vi "Main_FPGA.vi"() -> ()   [LabVIEW 2017]
uses:
  <vilib>/eio/EIONode/EIONode.xnode
  <vilib>/rvi/eio/common/nirviEmuTemplateMethod_errors.vi
  <vilib>/rvi/DataTransferAndStorage/Container/XNode/niFpgaContainer.xnode
  <vilib>/rvi/interface/RandomDataEmulation/nirviRandomDataFpgaMultiElementTemplate.vi
  <vilib>/eio/EIOPropertyNode/EIOPropertyNode.xnode
  <vilib>/rvi/eio/common/nirviEmuTemplatePropertyGet_errors.vi
  <vilib>/rvi/eio/common/nirviEmuTemplatePropertyGet_noerrors.vi
  <vilib>/rvi/eio/common/nirviEmuTemplatePropertySet_errors.vi
  <vilib>/rvi/eio/common/nirviEmuTemplatePropertySet_noerrors.vi
  <vilib>/eio/EIOMethodNode/EIOMethodNode.xnode
  <vilib>/LabVIEW Targets/FPGA/cRIO/shared/nicrio_ModuleControls/nicrio_cRIO-9770_DataRatesRing.ctl
panel:
  out "Chassis Temperature":sgl
  in  "Tab Control":T1(tab)
  out "Data Over-Run 1":bool
  out "Error 1":errorcluster
  out "LO Frequency (Hz) 1":u32
  out "Downconverter Gain (dB) 1":fxp<+/-,15,8>
  out "PeakRFPower 1":fxp<+/-,12,8>
  in  "AcqSettings.Ch 1":T3={"Center Frequency (Hz)"=10000000, "Data Rate"=0, "Number of Samples"=1000, "Continuous"=FALSE, "Reference Level (dBm)"=0.0} {"Data Rate" items=["320.000 kS/s (NI 9770)", "256.000 kS/s (NI 9770)", "128.000 kS/s (NI 9770)", "64.000 kS/s (NI 9770)", "32.000 kS/s (NI 9770)", "16.000 kS/s (NI 9770)", "8.000 kS/s (NI 9770)", "4.000 kS/s (NI 9770)"]; "Center Frequency (Hz)" format="%.0p"}
  in  "Start 1":bool
  in  "Stop 1":bool
  in  "Start 2":bool
  in  "AcqSettings.Ch 2":T3={"Center Frequency (Hz)"=10000000, "Data Rate"=0, "Number of Samples"=1000, "Continuous"=FALSE, "Reference Level (dBm)"=0.0} {"Data Rate" items=["320.000 kS/s (NI 9770)", "256.000 kS/s (NI 9770)", "128.000 kS/s (NI 9770)", "64.000 kS/s (NI 9770)", "32.000 kS/s (NI 9770)", "16.000 kS/s (NI 9770)", "8.000 kS/s (NI 9770)", "4.000 kS/s (NI 9770)"]; "Center Frequency (Hz)" format="%.0p"}
  out "PeakRFPower 2":fxp<+/-,12,8>
  out "Data Over-Run 2":bool
  in  "Stop 2":bool
  out "Error 2":errorcluster
  out "LO Frequency (Hz) 2":u32
  out "Downconverter Gain (dB) 2":fxp<+/-,15,8>
  in  "Start 3":bool
  in  "AcqSettings.Ch 3":T3={"Center Frequency (Hz)"=10000000, "Data Rate"=0, "Number of Samples"=1000, "Continuous"=FALSE, "Reference Level (dBm)"=0.0} {"Data Rate" items=["320.000 kS/s (NI 9770)", "256.000 kS/s (NI 9770)", "128.000 kS/s (NI 9770)", "64.000 kS/s (NI 9770)", "32.000 kS/s (NI 9770)", "16.000 kS/s (NI 9770)", "8.000 kS/s (NI 9770)", "4.000 kS/s (NI 9770)"]; "Center Frequency (Hz)" format="%.0p"}
  out "PeakRFPower 3":fxp<+/-,12,8>
  out "Data Over-Run 3":bool
  in  "Stop 3":bool
  out "Error 3":errorcluster
  out "LO Frequency (Hz) 3":u32
  out "Downconverter Gain (dB) 3":fxp<+/-,15,8>
  in  "Start 4":bool
  in  "AcqSettings.Ch 4":T3={"Center Frequency (Hz)"=10000000, "Data Rate"=0, "Number of Samples"=1000, "Continuous"=FALSE, "Reference Level (dBm)"=0.0} {"Data Rate" items=["320.000 kS/s (NI 9770)", "256.000 kS/s (NI 9770)", "128.000 kS/s (NI 9770)", "64.000 kS/s (NI 9770)", "32.000 kS/s (NI 9770)", "16.000 kS/s (NI 9770)", "8.000 kS/s (NI 9770)", "4.000 kS/s (NI 9770)"]; "Center Frequency (Hz)" format="%.0p"}
  out "PeakRFPower 4":fxp<+/-,12,8>
  out "Data Over-Run 4":bool
  in  "Stop 4":bool
  out "Error 4":errorcluster
  out "LO Frequency (Hz) 4":u32
  out "Downconverter Gain (dB) 4":fxp<+/-,15,8>
  in  "Start 5":bool
  in  "AcqSettings.Ch 5":T3={"Center Frequency (Hz)"=10000000, "Data Rate"=0, "Number of Samples"=1000, "Continuous"=FALSE, "Reference Level (dBm)"=0.0} {"Data Rate" items=["320.000 kS/s (NI 9770)", "256.000 kS/s (NI 9770)", "128.000 kS/s (NI 9770)", "64.000 kS/s (NI 9770)", "32.000 kS/s (NI 9770)", "16.000 kS/s (NI 9770)", "8.000 kS/s (NI 9770)", "4.000 kS/s (NI 9770)"]; "Center Frequency (Hz)" format="%.0p"}
  out "PeakRFPower 5":fxp<+/-,12,8>
  out "Data Over-Run 5":bool
  in  "Stop 5":bool
  out "Error 5":errorcluster
  out "LO Frequency (Hz) 5":u32
  out "Downconverter Gain (dB) 5":fxp<+/-,15,8>
  in  "Start 6":bool
  in  "AcqSettings.Ch 6":T3={"Center Frequency (Hz)"=10000000, "Data Rate"=0, "Number of Samples"=1000, "Continuous"=FALSE, "Reference Level (dBm)"=0.0} {"Data Rate" items=["320.000 kS/s (NI 9770)", "256.000 kS/s (NI 9770)", "128.000 kS/s (NI 9770)", "64.000 kS/s (NI 9770)", "32.000 kS/s (NI 9770)", "16.000 kS/s (NI 9770)", "8.000 kS/s (NI 9770)", "4.000 kS/s (NI 9770)"]; "Center Frequency (Hz)" format="%.0p"}
  out "PeakRFPower 6":fxp<+/-,12,8>
  out "Data Over-Run 6":bool
  in  "Stop 6":bool
  out "Error 6":errorcluster
  out "LO Frequency (Hz) 6":u32
  out "Downconverter Gain (dB) 6":fxp<+/-,15,8>
  in  "Start 7":bool
  in  "AcqSettings.Ch 7":T3={"Center Frequency (Hz)"=10000000, "Data Rate"=0, "Number of Samples"=1000, "Continuous"=FALSE, "Reference Level (dBm)"=0.0} {"Data Rate" items=["320.000 kS/s (NI 9770)", "256.000 kS/s (NI 9770)", "128.000 kS/s (NI 9770)", "64.000 kS/s (NI 9770)", "32.000 kS/s (NI 9770)", "16.000 kS/s (NI 9770)", "8.000 kS/s (NI 9770)", "4.000 kS/s (NI 9770)"]; "Center Frequency (Hz)" format="%.0p"}
  out "PeakRFPower 7":fxp<+/-,12,8>
  out "Data Over-Run 7":bool
  in  "Stop 7":bool
  out "Error 7":errorcluster
  out "LO Frequency (Hz) 7":u32
  out "Downconverter Gain (dB) 7":fxp<+/-,15,8>
  in  "Start 8":bool
  in  "AcqSettings.Ch 8":T3={"Center Frequency (Hz)"=10000000, "Data Rate"=0, "Number of Samples"=1000, "Continuous"=FALSE, "Reference Level (dBm)"=0.0} {"Data Rate" items=["320.000 kS/s (NI 9770)", "256.000 kS/s (NI 9770)", "128.000 kS/s (NI 9770)", "64.000 kS/s (NI 9770)", "32.000 kS/s (NI 9770)", "16.000 kS/s (NI 9770)", "8.000 kS/s (NI 9770)", "4.000 kS/s (NI 9770)"]; "Center Frequency (Hz)" format="%.0p"}
  out "PeakRFPower 8":fxp<+/-,12,8>
  out "Data Over-Run 8":bool
  in  "Stop 8":bool
  out "Error 8":errorcluster
  out "LO Frequency (Hz) 8":u32
  out "Downconverter Gain (dB) 8":fxp<+/-,15,8>
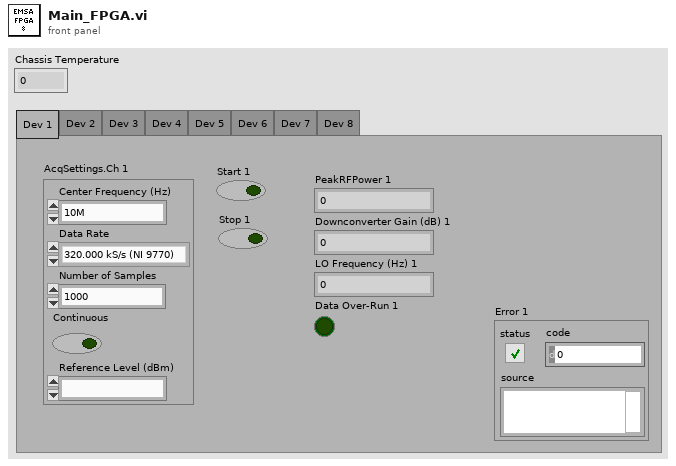
[diagram p1: front panel]
types:
  T1 = enum32{"Dev 1", "Dev 2", "Dev 3", "Dev 4", "Dev 5", "Dev 6", "Dev 7", "Dev 8"}
  T2 = typedef "nicrio_cRIO-9770_DataRatesRing.ctl" = u8
  T3 = cluster{"Center Frequency (Hz)":u32, "Data Rate":T2, "Number of Samples":i32, "Continuous":bool, "Reference Level (dBm)":fxp<+/-,14,7>}
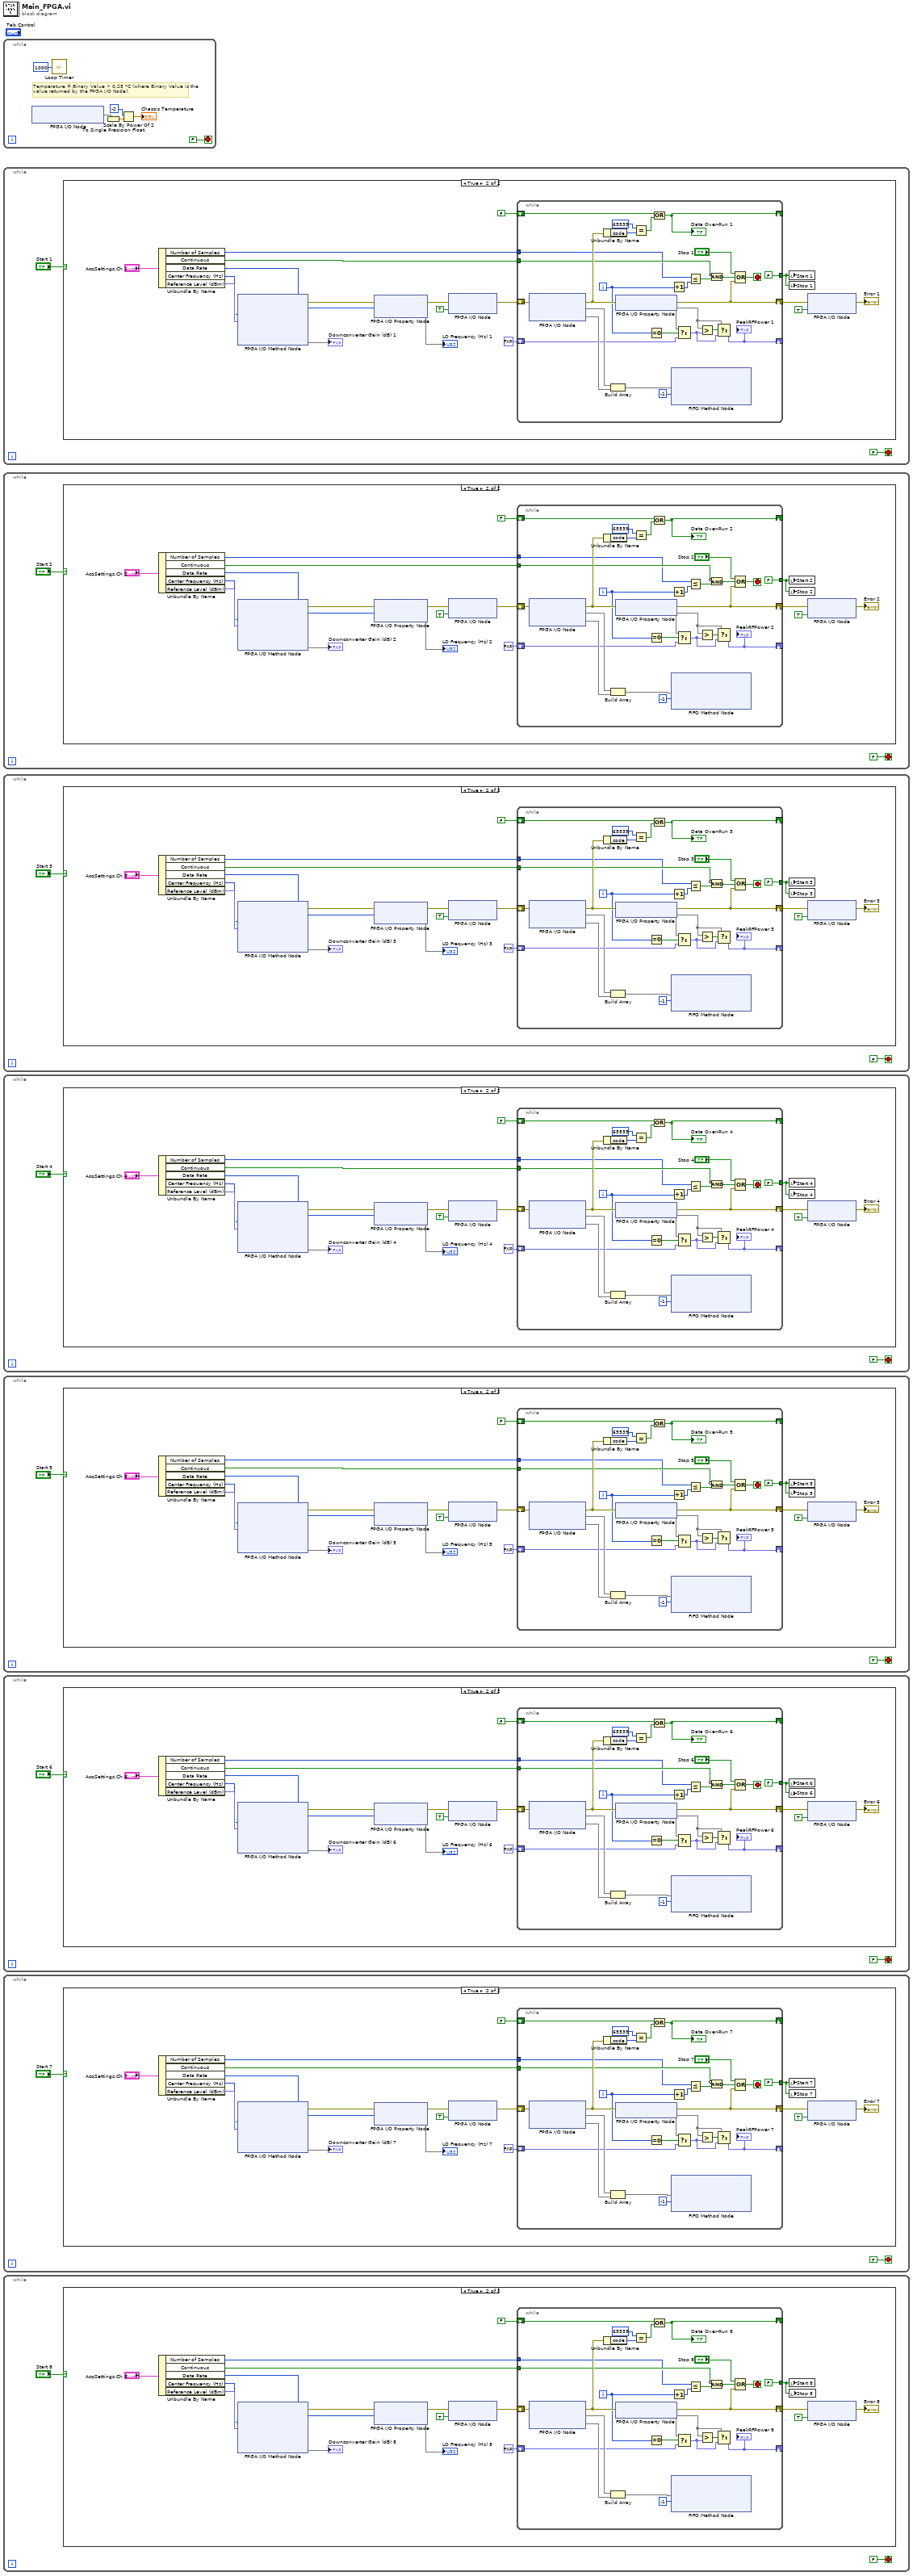
[diagram p0: block diagram]
diagram:
  n1 = while {
    stop <- FALSE stop-if-true
    # "Temperature = Binary Value × 0.25 °C (where Binary Value is the value returned by the FPGA I/O Node)."
    n2 = xnode "FPGA I/O Node"() -> ("Chassis Temperature"=w4)  [unwired: 1 in, 1 out]
    n3 = call "Loop Timer"("Count(mSec)"=u32 1000) -> ()  [unwired: 1 out]
    n4 = To Single Precision Float(number=w4) -> (single precision float=w6:sgl)
    n5 = Scale By Power Of 2(n=i16 -2, x=w6) -> (x*2^n=→"Chassis Temperature":sgl)
  }
  n6 = while {
    stop <- FALSE stop-if-true
    n7 = case shown="True" "Start 1" {
      frame False {
      }
      frame True {
        n8 = Unbundle By Name("AcqSettings.Ch 1") -> ("Number of Samples"=w10:i32, "Continuous"=w14:bool, "Data Rate"=w13:T2, "Center Frequency (Hz)"=w15:u32, "Reference Level (dBm)"=w16:fxp<+/-,14,7>)
        n9 = xnode "FPGA I/O Method Node"("Center Frequency"=w15, "Reference Level"=w16) -> ("error out"=w20:errorcluster, "Downconverter Gain"=→"Downconverter Gain (dB) 1")  [unwired: 4 in, 1 out]
        n10 = xnode "FPGA I/O Property Node"("error in"=w20, "Data Rate"=w13) -> ("error out"=w22:errorcluster, "LO Frequency"=→"LO Frequency (Hz) 1")  [unwired: 1 in, 1 out]
        n11 = xnode "FPGA I/O Node"("error in"=w22, "Mod1/Start"=TRUE ("start")) -> ("error out"=w21:errorcluster)  [unwired: 1 in, 1 out]
        n12 = while {
          shift-right: [w45] -> w25
          shift-left: w21 -> [w53]
          tunnel: [FALSE] -> w9
          shift-right: [w38] -> _
          shift-left: FALSE ("stop") -> [w40]
          shift-right: [w36] -> _
          shift-left: fxp<+/-,12,8> 0.0 ("Peak RF In Power") -> [w29]
          tunnel: w14 -> [w33]
          tunnel: w10 -> [w27]
          i -> [w31]
          stop <- w46 stop-if-true
          n13 = xnode "FPGA I/O Node"("error in"=w53) -> ("error out"=w43:errorcluster, "Mod1/RF In/I"=w52, "Mod1/RF In/Q"=w51)  [unwired: 2 in, 2 out]
          n14 = Unbundle By Name(w43) -> ("code"=w42:i32)
          n15 = Build Array(w52, w51) -> (w50:void[])
          n16 = xnode "FPGA I/O Property Node"("error in"=w43) -> ("error out"=w45:errorcluster, "Peak RF In Power"=w30)  [unwired: 1 in, 1 out]
          n17 = Equal?(x=65539, y=w42) -> (x = y?=w39:bool)
          n18 = Equal To 0?(x=w31) -> (x = 0?=w32:bool)
          n19 = Compound Arithmetic op=OR(w40, w39) -> (w38:bool)
          "Data Over-Run 1" <- w38
          n20 = xnode ("FIFO Method Node")("Element"=w50, "Timeout"=-1) -> ()  [unwired: 1 in, 2 out]
          n21 = Increment(x=w31) -> (x+1=w48:i32)
          n22 = Select(t=w30, s=w32, f=w29) -> (s? t:f=w28:fxp<+/-,12,8>)
          n23 = Less Or Equal?(x=w27, y=w48) -> (x <= y?=w35:bool)
          n24 = Greater?(x=w30, y=w28) -> (0:w37:bool)
          n25 = Compound Arithmetic op=AND(invert w33, w35) -> (w34:bool)
          n26 = Select(t=w30, s=w37, f=w28) -> (s? t:f=w36:fxp<+/-,12,8>)
          "PeakRFPower 1" <- w36
          n27 = Compound Arithmetic op=OR("Stop 1", w34, w45) -> (w46:bool)
        }
        n28 = local write "Start 1"(w9) -> ()
        n29 = local write "Stop 1"(w9) -> ()
        n30 = xnode "FPGA I/O Node"("error in"=w25, "Mod1/Stop"=TRUE ("stop")) -> ("error out"=→"Error 1":errorcluster)  [unwired: 1 in, 1 out]
      }
    }
  }
  n31 = while {
    stop <- FALSE stop-if-true
    n32 = case shown="True" "Start 2" {
      frame False {
      }
      frame True {
        n33 = Unbundle By Name("AcqSettings.Ch 2") -> ("Number of Samples"=w57:i32, "Continuous"=w61:bool, "Data Rate"=w60:T2, "Center Frequency (Hz)"=w62:u32, "Reference Level (dBm)"=w63:fxp<+/-,14,7>)
        n34 = xnode "FPGA I/O Method Node"("Center Frequency"=w62, "Reference Level"=w63) -> ("error out"=w67:errorcluster, "Downconverter Gain"=→"Downconverter Gain (dB) 2")  [unwired: 4 in, 1 out]
        n35 = xnode "FPGA I/O Property Node"("error in"=w67, "Data Rate"=w60) -> ("error out"=w69:errorcluster, "LO Frequency"=→"LO Frequency (Hz) 2")  [unwired: 1 in, 1 out]
        n36 = xnode "FPGA I/O Node"("error in"=w69, "Mod2/Start"=TRUE ("start")) -> ("error out"=w68:errorcluster)  [unwired: 1 in, 1 out]
        n37 = while {
          shift-right: [w92] -> w72
          shift-left: w68 -> [w100]
          tunnel: [FALSE] -> w56
          shift-right: [w85] -> _
          shift-left: FALSE ("stop") -> [w87]
          shift-right: [w83] -> _
          shift-left: fxp<+/-,12,8> 0.0 ("Peak RF In Power") -> [w76]
          tunnel: w61 -> [w80]
          tunnel: w57 -> [w74]
          i -> [w78]
          stop <- w93 stop-if-true
          n38 = xnode "FPGA I/O Node"("error in"=w100) -> ("error out"=w90:errorcluster, "Mod2/RF In/I"=w99, "Mod2/RF In/Q"=w98)  [unwired: 2 in, 2 out]
          n39 = Unbundle By Name(w90) -> ("code"=w89:i32)
          n40 = Build Array(w99, w98) -> (w97:void[])
          n41 = xnode "FPGA I/O Property Node"("error in"=w90) -> ("error out"=w92:errorcluster, "Peak RF In Power"=w77)  [unwired: 1 in, 1 out]
          n42 = Equal?(x=65539, y=w89) -> (x = y?=w86:bool)
          n43 = Equal To 0?(x=w78) -> (x = 0?=w79:bool)
          n44 = Compound Arithmetic op=OR(w87, w86) -> (w85:bool)
          "Data Over-Run 2" <- w85
          n45 = xnode ("FIFO Method Node")("Element"=w97, "Timeout"=-1) -> ()  [unwired: 1 in, 2 out]
          n46 = Increment(x=w78) -> (x+1=w95:i32)
          n47 = Select(t=w77, s=w79, f=w76) -> (s? t:f=w75:fxp<+/-,12,8>)
          n48 = Less Or Equal?(x=w74, y=w95) -> (x <= y?=w82:bool)
          n49 = Greater?(x=w77, y=w75) -> (0:w84:bool)
          n50 = Compound Arithmetic op=AND(invert w80, w82) -> (w81:bool)
          n51 = Select(t=w77, s=w84, f=w75) -> (s? t:f=w83:fxp<+/-,12,8>)
          "PeakRFPower 2" <- w83
          n52 = Compound Arithmetic op=OR("Stop 2", w81, w92) -> (w93:bool)
        }
        n53 = local write "Start 2"(w56) -> ()
        n54 = local write "Stop 2"(w56) -> ()
        n55 = xnode "FPGA I/O Node"("error in"=w72, "Mod2/Stop"=TRUE ("stop")) -> ("error out"=→"Error 2":errorcluster)  [unwired: 1 in, 1 out]
      }
    }
  }
  n56 = while {
    stop <- FALSE stop-if-true
    n57 = case shown="True" "Start 3" {
      frame False {
      }
      frame True {
        n58 = Unbundle By Name("AcqSettings.Ch 3") -> ("Number of Samples"=w104:i32, "Continuous"=w108:bool, "Data Rate"=w107:T2, "Center Frequency (Hz)"=w109:u32, "Reference Level (dBm)"=w110:fxp<+/-,14,7>)
        n59 = xnode "FPGA I/O Method Node"("Center Frequency"=w109, "Reference Level"=w110) -> ("error out"=w114:errorcluster, "Downconverter Gain"=→"Downconverter Gain (dB) 3")  [unwired: 4 in, 1 out]
        n60 = xnode "FPGA I/O Property Node"("error in"=w114, "Data Rate"=w107) -> ("error out"=w116:errorcluster, "LO Frequency"=→"LO Frequency (Hz) 3")  [unwired: 1 in, 1 out]
        n61 = xnode "FPGA I/O Node"("error in"=w116, "Mod3/Start"=TRUE ("start")) -> ("error out"=w115:errorcluster)  [unwired: 1 in, 1 out]
        n62 = while {
          shift-right: [w139] -> w119
          shift-left: w115 -> [w147]
          tunnel: [FALSE] -> w103
          shift-right: [w132] -> _
          shift-left: FALSE ("stop") -> [w134]
          shift-right: [w130] -> _
          shift-left: fxp<+/-,12,8> 0.0 ("Peak RF In Power") -> [w123]
          tunnel: w108 -> [w127]
          tunnel: w104 -> [w121]
          i -> [w125]
          stop <- w140 stop-if-true
          n63 = xnode "FPGA I/O Node"("error in"=w147) -> ("error out"=w137:errorcluster, "Mod3/RF In/I"=w146, "Mod3/RF In/Q"=w145)  [unwired: 2 in, 2 out]
          n64 = Unbundle By Name(w137) -> ("code"=w136:i32)
          n65 = Build Array(w146, w145) -> (w144:void[])
          n66 = xnode "FPGA I/O Property Node"("error in"=w137) -> ("error out"=w139:errorcluster, "Peak RF In Power"=w124)  [unwired: 1 in, 1 out]
          n67 = Equal?(x=65539, y=w136) -> (x = y?=w133:bool)
          n68 = Equal To 0?(x=w125) -> (x = 0?=w126:bool)
          n69 = Compound Arithmetic op=OR(w134, w133) -> (w132:bool)
          "Data Over-Run 3" <- w132
          n70 = xnode ("FIFO Method Node")("Element"=w144, "Timeout"=-1) -> ()  [unwired: 1 in, 2 out]
          n71 = Increment(x=w125) -> (x+1=w142:i32)
          n72 = Select(t=w124, s=w126, f=w123) -> (s? t:f=w122:fxp<+/-,12,8>)
          n73 = Less Or Equal?(x=w121, y=w142) -> (x <= y?=w129:bool)
          n74 = Greater?(x=w124, y=w122) -> (0:w131:bool)
          n75 = Compound Arithmetic op=AND(invert w127, w129) -> (w128:bool)
          n76 = Select(t=w124, s=w131, f=w122) -> (s? t:f=w130:fxp<+/-,12,8>)
          "PeakRFPower 3" <- w130
          n77 = Compound Arithmetic op=OR("Stop 3", w128, w139) -> (w140:bool)
        }
        n78 = local write "Start 3"(w103) -> ()
        n79 = local write "Stop 3"(w103) -> ()
        n80 = xnode "FPGA I/O Node"("error in"=w119, "Mod3/Stop"=TRUE ("stop")) -> ("error out"=→"Error 3":errorcluster)  [unwired: 1 in, 1 out]
      }
    }
  }
  n81 = while {
    stop <- FALSE stop-if-true
    n82 = case shown="True" "Start 4" {
      frame False {
      }
      frame True {
        n83 = Unbundle By Name("AcqSettings.Ch 4") -> ("Number of Samples"=w151:i32, "Continuous"=w155:bool, "Data Rate"=w154:T2, "Center Frequency (Hz)"=w156:u32, "Reference Level (dBm)"=w157:fxp<+/-,14,7>)
        n84 = xnode "FPGA I/O Method Node"("Center Frequency"=w156, "Reference Level"=w157) -> ("error out"=w161:errorcluster, "Downconverter Gain"=→"Downconverter Gain (dB) 4")  [unwired: 4 in, 1 out]
        n85 = xnode "FPGA I/O Property Node"("error in"=w161, "Data Rate"=w154) -> ("error out"=w163:errorcluster, "LO Frequency"=→"LO Frequency (Hz) 4")  [unwired: 1 in, 1 out]
        n86 = xnode "FPGA I/O Node"("error in"=w163, "Mod4/Start"=TRUE ("start")) -> ("error out"=w162:errorcluster)  [unwired: 1 in, 1 out]
        n87 = while {
          shift-right: [w186] -> w166
          shift-left: w162 -> [w194]
          tunnel: [FALSE] -> w150
          shift-right: [w179] -> _
          shift-left: FALSE ("stop") -> [w181]
          shift-right: [w177] -> _
          shift-left: fxp<+/-,12,8> 0.0 ("Peak RF In Power") -> [w170]
          tunnel: w155 -> [w174]
          tunnel: w151 -> [w168]
          i -> [w172]
          stop <- w187 stop-if-true
          n88 = xnode "FPGA I/O Node"("error in"=w194) -> ("error out"=w184:errorcluster, "Mod4/RF In/I"=w193, "Mod4/RF In/Q"=w192)  [unwired: 2 in, 2 out]
          n89 = Unbundle By Name(w184) -> ("code"=w183:i32)
          n90 = Build Array(w193, w192) -> (w191:void[])
          n91 = xnode "FPGA I/O Property Node"("error in"=w184) -> ("error out"=w186:errorcluster, "Peak RF In Power"=w171)  [unwired: 1 in, 1 out]
          n92 = Equal?(x=65539, y=w183) -> (x = y?=w180:bool)
          n93 = Equal To 0?(x=w172) -> (x = 0?=w173:bool)
          n94 = Compound Arithmetic op=OR(w181, w180) -> (w179:bool)
          "Data Over-Run 4" <- w179
          n95 = xnode ("FIFO Method Node")("Element"=w191, "Timeout"=-1) -> ()  [unwired: 1 in, 2 out]
          n96 = Increment(x=w172) -> (x+1=w189:i32)
          n97 = Select(t=w171, s=w173, f=w170) -> (s? t:f=w169:fxp<+/-,12,8>)
          n98 = Less Or Equal?(x=w168, y=w189) -> (x <= y?=w176:bool)
          n99 = Greater?(x=w171, y=w169) -> (0:w178:bool)
          n100 = Compound Arithmetic op=AND(invert w174, w176) -> (w175:bool)
          n101 = Select(t=w171, s=w178, f=w169) -> (s? t:f=w177:fxp<+/-,12,8>)
          "PeakRFPower 4" <- w177
          n102 = Compound Arithmetic op=OR("Stop 4", w175, w186) -> (w187:bool)
        }
        n103 = local write "Start 4"(w150) -> ()
        n104 = local write "Stop 4"(w150) -> ()
        n105 = xnode "FPGA I/O Node"("error in"=w166, "Mod4/Stop"=TRUE ("stop")) -> ("error out"=→"Error 4":errorcluster)  [unwired: 1 in, 1 out]
      }
    }
  }
  n106 = while {
    stop <- FALSE stop-if-true
    n107 = case shown="True" "Start 5" {
      frame False {
      }
      frame True {
        n108 = Unbundle By Name("AcqSettings.Ch 5") -> ("Number of Samples"=w198:i32, "Continuous"=w202:bool, "Data Rate"=w201:T2, "Center Frequency (Hz)"=w203:u32, "Reference Level (dBm)"=w204:fxp<+/-,14,7>)
        n109 = xnode "FPGA I/O Method Node"("Center Frequency"=w203, "Reference Level"=w204) -> ("error out"=w208:errorcluster, "Downconverter Gain"=→"Downconverter Gain (dB) 5")  [unwired: 4 in, 1 out]
        n110 = xnode "FPGA I/O Property Node"("error in"=w208, "Data Rate"=w201) -> ("error out"=w210:errorcluster, "LO Frequency"=→"LO Frequency (Hz) 5")  [unwired: 1 in, 1 out]
        n111 = xnode "FPGA I/O Node"("error in"=w210, "Mod5/Start"=TRUE ("start")) -> ("error out"=w209:errorcluster)  [unwired: 1 in, 1 out]
        n112 = while {
          shift-right: [w233] -> w213
          shift-left: w209 -> [w241]
          tunnel: [FALSE] -> w197
          shift-right: [w226] -> _
          shift-left: FALSE ("stop") -> [w228]
          shift-right: [w224] -> _
          shift-left: fxp<+/-,12,8> 0.0 ("Peak RF In Power") -> [w217]
          tunnel: w202 -> [w221]
          tunnel: w198 -> [w215]
          i -> [w219]
          stop <- w234 stop-if-true
          n113 = xnode "FPGA I/O Node"("error in"=w241) -> ("error out"=w231:errorcluster, "Mod5/RF In/I"=w240, "Mod5/RF In/Q"=w239)  [unwired: 2 in, 2 out]
          n114 = Unbundle By Name(w231) -> ("code"=w230:i32)
          n115 = Build Array(w240, w239) -> (w238:void[])
          n116 = xnode "FPGA I/O Property Node"("error in"=w231) -> ("error out"=w233:errorcluster, "Peak RF In Power"=w218)  [unwired: 1 in, 1 out]
          n117 = Equal?(x=65539, y=w230) -> (x = y?=w227:bool)
          n118 = Equal To 0?(x=w219) -> (x = 0?=w220:bool)
          n119 = Compound Arithmetic op=OR(w228, w227) -> (w226:bool)
          "Data Over-Run 5" <- w226
          n120 = xnode ("FIFO Method Node")("Element"=w238, "Timeout"=-1) -> ()  [unwired: 1 in, 2 out]
          n121 = Increment(x=w219) -> (x+1=w236:i32)
          n122 = Select(t=w218, s=w220, f=w217) -> (s? t:f=w216:fxp<+/-,12,8>)
          n123 = Less Or Equal?(x=w215, y=w236) -> (x <= y?=w223:bool)
          n124 = Greater?(x=w218, y=w216) -> (0:w225:bool)
          n125 = Compound Arithmetic op=AND(invert w221, w223) -> (w222:bool)
          n126 = Select(t=w218, s=w225, f=w216) -> (s? t:f=w224:fxp<+/-,12,8>)
          "PeakRFPower 5" <- w224
          n127 = Compound Arithmetic op=OR("Stop 5", w222, w233) -> (w234:bool)
        }
        n128 = local write "Start 5"(w197) -> ()
        n129 = local write "Stop 5"(w197) -> ()
        n130 = xnode "FPGA I/O Node"("error in"=w213, "Mod5/Stop"=TRUE ("stop")) -> ("error out"=→"Error 5":errorcluster)  [unwired: 1 in, 1 out]
      }
    }
  }
  n131 = while {
    stop <- FALSE stop-if-true
    n132 = case shown="True" "Start 6" {
      frame False {
      }
      frame True {
        n133 = Unbundle By Name("AcqSettings.Ch 6") -> ("Number of Samples"=w245:i32, "Continuous"=w249:bool, "Data Rate"=w248:T2, "Center Frequency (Hz)"=w250:u32, "Reference Level (dBm)"=w251:fxp<+/-,14,7>)
        n134 = xnode "FPGA I/O Method Node"("Center Frequency"=w250, "Reference Level"=w251) -> ("error out"=w255:errorcluster, "Downconverter Gain"=→"Downconverter Gain (dB) 6")  [unwired: 4 in, 1 out]
        n135 = xnode "FPGA I/O Property Node"("error in"=w255, "Data Rate"=w248) -> ("error out"=w257:errorcluster, "LO Frequency"=→"LO Frequency (Hz) 6")  [unwired: 1 in, 1 out]
        n136 = xnode "FPGA I/O Node"("error in"=w257, "Mod6/Start"=TRUE ("start")) -> ("error out"=w256:errorcluster)  [unwired: 1 in, 1 out]
        n137 = while {
          shift-right: [w280] -> w260
          shift-left: w256 -> [w288]
          tunnel: [FALSE] -> w244
          shift-right: [w273] -> _
          shift-left: FALSE ("stop") -> [w275]
          shift-right: [w271] -> _
          shift-left: fxp<+/-,12,8> 0.0 ("Peak RF In Power") -> [w264]
          tunnel: w249 -> [w268]
          tunnel: w245 -> [w262]
          i -> [w266]
          stop <- w281 stop-if-true
          n138 = xnode "FPGA I/O Node"("error in"=w288) -> ("error out"=w278:errorcluster, "Mod6/RF In/I"=w287, "Mod6/RF In/Q"=w286)  [unwired: 2 in, 2 out]
          n139 = Unbundle By Name(w278) -> ("code"=w277:i32)
          n140 = Build Array(w287, w286) -> (w285:void[])
          n141 = xnode "FPGA I/O Property Node"("error in"=w278) -> ("error out"=w280:errorcluster, "Peak RF In Power"=w265)  [unwired: 1 in, 1 out]
          n142 = Equal?(x=65539, y=w277) -> (x = y?=w274:bool)
          n143 = Equal To 0?(x=w266) -> (x = 0?=w267:bool)
          n144 = Compound Arithmetic op=OR(w275, w274) -> (w273:bool)
          "Data Over-Run 6" <- w273
          n145 = xnode ("FIFO Method Node")("Element"=w285, "Timeout"=-1) -> ()  [unwired: 1 in, 2 out]
          n146 = Increment(x=w266) -> (x+1=w283:i32)
          n147 = Select(t=w265, s=w267, f=w264) -> (s? t:f=w263:fxp<+/-,12,8>)
          n148 = Less Or Equal?(x=w262, y=w283) -> (x <= y?=w270:bool)
          n149 = Greater?(x=w265, y=w263) -> (0:w272:bool)
          n150 = Compound Arithmetic op=AND(invert w268, w270) -> (w269:bool)
          n151 = Select(t=w265, s=w272, f=w263) -> (s? t:f=w271:fxp<+/-,12,8>)
          "PeakRFPower 6" <- w271
          n152 = Compound Arithmetic op=OR("Stop 6", w269, w280) -> (w281:bool)
        }
        n153 = local write "Start 6"(w244) -> ()
        n154 = local write "Stop 6"(w244) -> ()
        n155 = xnode "FPGA I/O Node"("error in"=w260, "Mod6/Stop"=TRUE ("stop")) -> ("error out"=→"Error 6":errorcluster)  [unwired: 1 in, 1 out]
      }
    }
  }
  n156 = while {
    stop <- FALSE stop-if-true
    n157 = case shown="True" "Start 7" {
      frame False {
      }
      frame True {
        n158 = Unbundle By Name("AcqSettings.Ch 7") -> ("Number of Samples"=w292:i32, "Continuous"=w296:bool, "Data Rate"=w295:T2, "Center Frequency (Hz)"=w297:u32, "Reference Level (dBm)"=w298:fxp<+/-,14,7>)
        n159 = xnode "FPGA I/O Method Node"("Center Frequency"=w297, "Reference Level"=w298) -> ("error out"=w302:errorcluster, "Downconverter Gain"=→"Downconverter Gain (dB) 7")  [unwired: 4 in, 1 out]
        n160 = xnode "FPGA I/O Property Node"("error in"=w302, "Data Rate"=w295) -> ("error out"=w304:errorcluster, "LO Frequency"=→"LO Frequency (Hz) 7")  [unwired: 1 in, 1 out]
        n161 = xnode "FPGA I/O Node"("error in"=w304, "Mod7/Start"=TRUE ("start")) -> ("error out"=w303:errorcluster)  [unwired: 1 in, 1 out]
        n162 = while {
          shift-right: [w327] -> w307
          shift-left: w303 -> [w335]
          tunnel: [FALSE] -> w291
          shift-right: [w320] -> _
          shift-left: FALSE ("stop") -> [w322]
          shift-right: [w318] -> _
          shift-left: fxp<+/-,12,8> 0.0 ("Peak RF In Power") -> [w311]
          tunnel: w296 -> [w315]
          tunnel: w292 -> [w309]
          i -> [w313]
          stop <- w328 stop-if-true
          n163 = xnode "FPGA I/O Node"("error in"=w335) -> ("error out"=w325:errorcluster, "Mod7/RF In/I"=w334, "Mod7/RF In/Q"=w333)  [unwired: 2 in, 2 out]
          n164 = Unbundle By Name(w325) -> ("code"=w324:i32)
          n165 = Build Array(w334, w333) -> (w332:void[])
          n166 = xnode "FPGA I/O Property Node"("error in"=w325) -> ("error out"=w327:errorcluster, "Peak RF In Power"=w312)  [unwired: 1 in, 1 out]
          n167 = Equal?(x=65539, y=w324) -> (x = y?=w321:bool)
          n168 = Equal To 0?(x=w313) -> (x = 0?=w314:bool)
          n169 = Compound Arithmetic op=OR(w322, w321) -> (w320:bool)
          "Data Over-Run 7" <- w320
          n170 = xnode ("FIFO Method Node")("Element"=w332, "Timeout"=-1) -> ()  [unwired: 1 in, 2 out]
          n171 = Increment(x=w313) -> (x+1=w330:i32)
          n172 = Select(t=w312, s=w314, f=w311) -> (s? t:f=w310:fxp<+/-,12,8>)
          n173 = Less Or Equal?(x=w309, y=w330) -> (x <= y?=w317:bool)
          n174 = Greater?(x=w312, y=w310) -> (0:w319:bool)
          n175 = Compound Arithmetic op=AND(invert w315, w317) -> (w316:bool)
          n176 = Select(t=w312, s=w319, f=w310) -> (s? t:f=w318:fxp<+/-,12,8>)
          "PeakRFPower 7" <- w318
          n177 = Compound Arithmetic op=OR("Stop 7", w316, w327) -> (w328:bool)
        }
        n178 = local write "Start 7"(w291) -> ()
        n179 = local write "Stop 7"(w291) -> ()
        n180 = xnode "FPGA I/O Node"("error in"=w307, "Mod7/Stop"=TRUE ("stop")) -> ("error out"=→"Error 7":errorcluster)  [unwired: 1 in, 1 out]
      }
    }
  }
  n181 = while {
    stop <- FALSE stop-if-true
    n182 = case shown="True" "Start 8" {
      frame False {
      }
      frame True {
        n183 = Unbundle By Name("AcqSettings.Ch 8") -> ("Number of Samples"=w339:i32, "Continuous"=w343:bool, "Data Rate"=w342:T2, "Center Frequency (Hz)"=w344:u32, "Reference Level (dBm)"=w345:fxp<+/-,14,7>)
        n184 = xnode "FPGA I/O Method Node"("Center Frequency"=w344, "Reference Level"=w345) -> ("error out"=w349:errorcluster, "Downconverter Gain"=→"Downconverter Gain (dB) 8")  [unwired: 4 in, 1 out]
        n185 = xnode "FPGA I/O Property Node"("error in"=w349, "Data Rate"=w342) -> ("error out"=w351:errorcluster, "LO Frequency"=→"LO Frequency (Hz) 8")  [unwired: 1 in, 1 out]
        n186 = xnode "FPGA I/O Node"("error in"=w351, "Mod8/Start"=TRUE ("start")) -> ("error out"=w350:errorcluster)  [unwired: 1 in, 1 out]
        n187 = while {
          shift-right: [w374] -> w354
          shift-left: w350 -> [w382]
          tunnel: [FALSE] -> w338
          shift-right: [w367] -> _
          shift-left: FALSE ("stop") -> [w369]
          shift-right: [w365] -> _
          shift-left: fxp<+/-,12,8> 0.0 ("Peak RF In Power") -> [w358]
          tunnel: w343 -> [w362]
          tunnel: w339 -> [w356]
          i -> [w360]
          stop <- w375 stop-if-true
          n188 = xnode "FPGA I/O Node"("error in"=w382) -> ("error out"=w372:errorcluster, "Mod8/RF In/I"=w381, "Mod8/RF In/Q"=w380)  [unwired: 2 in, 2 out]
          n189 = Unbundle By Name(w372) -> ("code"=w371:i32)
          n190 = Build Array(w381, w380) -> (w379:void[])
          n191 = xnode "FPGA I/O Property Node"("error in"=w372) -> ("error out"=w374:errorcluster, "Peak RF In Power"=w359)  [unwired: 1 in, 1 out]
          n192 = Equal?(x=65539, y=w371) -> (x = y?=w368:bool)
          n193 = Equal To 0?(x=w360) -> (x = 0?=w361:bool)
          n194 = Compound Arithmetic op=OR(w369, w368) -> (w367:bool)
          "Data Over-Run 8" <- w367
          n195 = xnode ("FIFO Method Node")("Element"=w379, "Timeout"=-1) -> ()  [unwired: 1 in, 2 out]
          n196 = Increment(x=w360) -> (x+1=w377:i32)
          n197 = Select(t=w359, s=w361, f=w358) -> (s? t:f=w357:fxp<+/-,12,8>)
          n198 = Less Or Equal?(x=w356, y=w377) -> (x <= y?=w364:bool)
          n199 = Greater?(x=w359, y=w357) -> (0:w366:bool)
          n200 = Compound Arithmetic op=AND(invert w362, w364) -> (w363:bool)
          n201 = Select(t=w359, s=w366, f=w357) -> (s? t:f=w365:fxp<+/-,12,8>)
          "PeakRFPower 8" <- w365
          n202 = Compound Arithmetic op=OR("Stop 8", w363, w374) -> (w375:bool)
        }
        n203 = local write "Start 8"(w338) -> ()
        n204 = local write "Stop 8"(w338) -> ()
        n205 = xnode "FPGA I/O Node"("error in"=w354, "Mod8/Stop"=TRUE ("stop")) -> ("error out"=→"Error 8":errorcluster)  [unwired: 1 in, 1 out]
      }
    }
  }
